vi "Run.vi"(8 "error in (no error)":errorcluster, 11 "MB in":refnum<class "WebSocket Client CR.lvclass">) -> (0 "error out":errorcluster, 3 "MB out":refnum<class "WebSocket Client CR.lvclass">)   [LabVIEW 2021, in "WebSockets.lvlib" / "WebSocket Client CR.lvclass"]
uses:
  WebSocket Client CR.lvclass
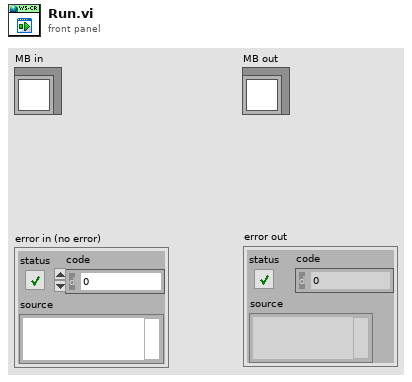
[diagram p1: front panel]
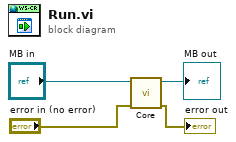
[diagram p0: block diagram]
diagram:
  n1 = call-dynamic "Core.vi"("error in (no error)"="error in (no error)", "MB in"="MB in") -> ("error out"=→"error out":errorcluster, "MB out"=→"MB out":refnum<class "WebSocket Client CR.lvclass">)  [unwired: 8 in]
